vi "Independent Commands.vi"(11 "Buttons":bool[](array[boolean])) -> ()   [LabVIEW 2018]
uses:
  0198bb7d-f57a-4b66-b85a-08a0d8482cc4.vi
  Robot Global Data.vi
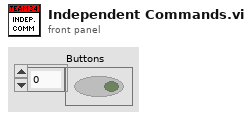
[diagram p1: front panel]
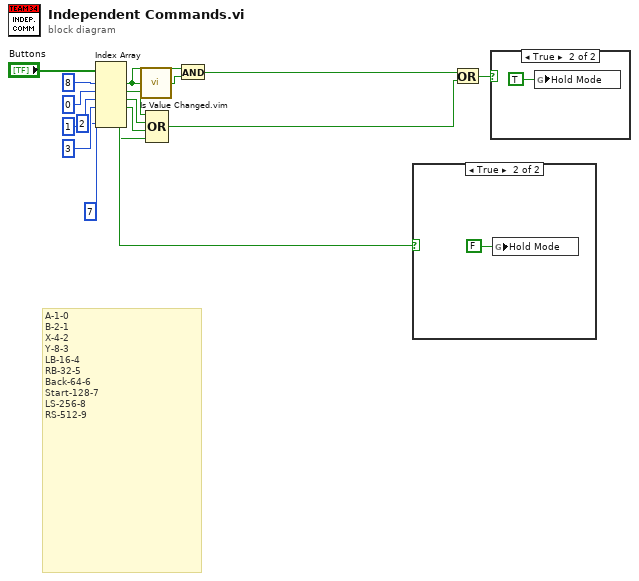
[diagram p0: block diagram]
diagram:
  # "A-1-0\nB-2-1\nX-4-2\nY-8-3\nLB-16-4\nRB-32-5\nBack-64-6\nStart-128-7\nLS-256-8\nRS-512-9"
  n1 = Index Array(array="Buttons", index #1=8 ("index"), index #2=0 ("index"), index #3=1 ("index"), index #4=3 ("index"), index #5=7 ("index"), index #6=2 ("index")) -> (element #1=w15:bool, element #2=w10:bool, element #3=w9:bool, element #4=w8:bool, element #5=w3:bool, element #6=w1:bool)
  n2 = call "Is Value Changed.vim"("value"=w15) -> ("changed or first call?"=w14:bool)
  n3 = Compound Arithmetic op=OR(w10, w9, w8, w1) -> (w5:bool)
  n4 = And(x=w15, y=w14) -> (x .and. y?=w7:bool)
  n5 = case shown="True" w3 {
    frame False {
    }
    frame True {
      n6 = global write "Robot Global Data.vi" "Hold Mode"(FALSE ("Hold Mode")) -> ()
    }
  }
  n7 = Or(x=w7, y=w5) -> (x .or. y?=w6:bool)
  n8 = case shown="True" w6 {
    frame False {
    }
    frame True {
      n9 = global write "Robot Global Data.vi" "Hold Mode"(TRUE ("Hold Mode")) -> ()
    }
  }
